vi "getMDBFile.vi"() -> ()   [LabVIEW 2012]
uses:
  <vilib>/addons/database/Auxilliary.llb/DB Tools Cursor Type.ctl
  <vilib>/addons/database/Connection.llb/DB Tools Open Connec (String).vi
  <vilib>/addons/database/Connection.llb/Conn Execute.vi
  <vilib>/addons/database/Recordset.llb/Rec Fetch Recordset Data (R).vi
  <vilib>/addons/database/Recordset.llb/Rec Destroy - Connection.vi
  <vilib>/addons/database/NI_Database_API.lvlib
panel:
  out "concatenated string 2":string
  out "recordset data":variant[][](array[variant])
  out "error out 2":errorcluster
  out "path out":path
  out "filenames":string[](array[string])
  in  "path":path
  out "concatenated string":string
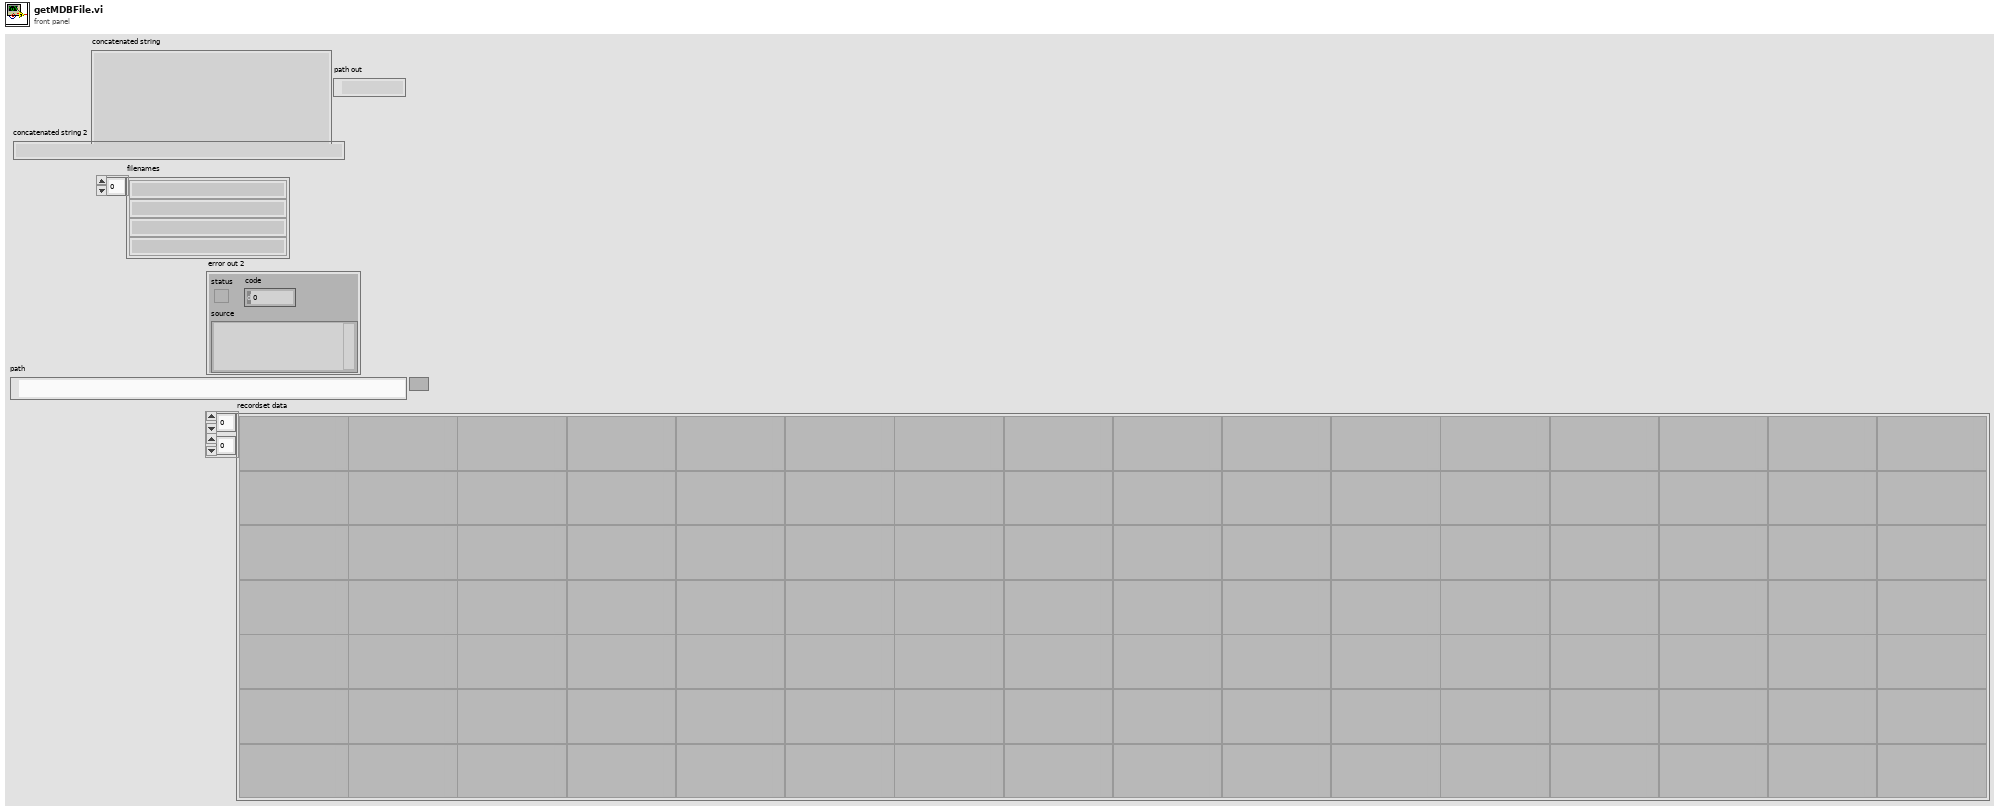
[diagram p1: front panel]
types:
  T1 = typedef "NI_Database_API.lvlib/DB Tools Cursor Type.ctl" = enum16{"forward-only", "keyset", "dynamic", "static"}
  T2 = typedef "NI_Database_API.lvlib/Conn ObjectReference.ctl" = refnum<k1>
  T3 = typedef "NI_Database_API.lvlib/Rec ObjectReference.ctl" = refnum<k1>
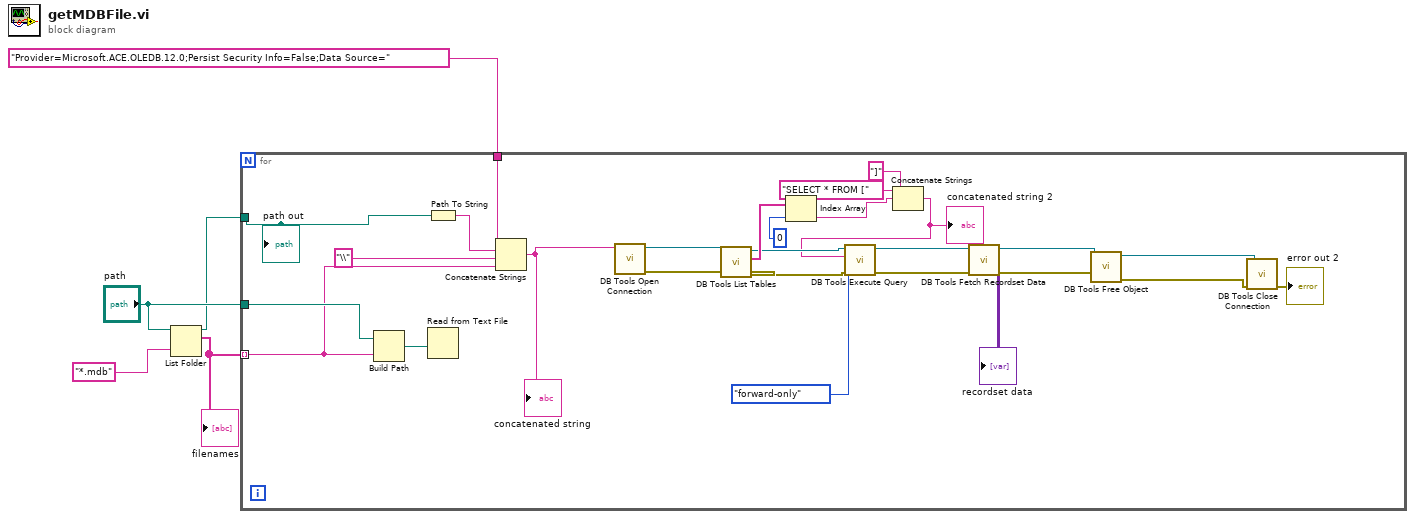
[diagram p0: block diagram]
diagram:
  n1 = List Folder(path="path", pattern="*.mdb") -> (path out=w1:path, filenames=w3:string[])  [unwired: 2 in, 2 out]
  "filenames" <- w3
  n2 = for {
    tunnel: "path" -> [w31]
    tunnel: w3 -> [w26] mode=indexing
    tunnel: "Provider=Microsoft.ACE.OLEDB.12.0;Persist Security Info=False;Data Source=" -> [w28]
    tunnel: w1 -> [w27]
    n3 = Build Path(base path=w31, name or relative path=w26) -> (appended path=w32:path)
    n4 = Path To String(path=w27) -> (string=w30:string)
    n5 = Read from Text File(file (use dialog)=w32) -> ()  [unwired: 3 in, 4 out]
    n6 = Concatenate Strings(w28, w30, "\\", w26) -> (w25:string)
    "concatenated string" <- w25
    n7 = call-poly <vilib>:"DB Tools Open Connection.vi"("connection information"=w25) -> ("error out"=w22:errorcluster, "connection reference"=w23:T2)  [unwired: 7 in]
    n8 = call <vilib>:"DB Tools List Tables.vi"("error in (no error)"=w22, "connection reference"=w23) -> ("error out"=w18:errorcluster, "tables"=w21:string[], "connection reference out"=w19:T2)  [unwired: 3 in]
    n9 = Index Array(array=w21, index=0) -> (element=w9:string)
    n10 = Concatenate Strings("SELECT * FROM [" ("string"), w9, "]" ("string")) -> (w8:string)
    "concatenated string 2" <- w8
    n11 = call-poly <vilib>:"DB Tools Execute Query.vi"("error in (no error)"=w18, "cursor type"=DB_Tools_Cursor_Type."forward-only", "SQL query"=w8, "connection reference"=w19) -> ("error out"=w16:errorcluster, "recordset reference"=w17:T3)  [unwired: 4 in]
    n12 = call-poly <vilib>:"DB Tools Fetch Recordset Data.vi"("error in (no error)"=w16, "recordset reference"=w17) -> ("error out"=w14:errorcluster, "recordset data"=→"recordset data":variant[][], "recordset reference out"=w15:T3)  [unwired: 3 in]
    n13 = call-poly <vilib>:"DB Tools Free Object.vi"("error in (no error)"=w14, "recordset reference"=w15) -> ("error out"=w12:errorcluster, "connection reference"=w13:T2)  [unwired: 8 in]
    n14 = call <vilib>:"DB Tools Close Connection.vi"("error in (no error)"=w12, "connection reference"=w13) -> ("error out"=→"error out 2":errorcluster)  [unwired: 5 in]
    "path out" <- w27
  }
